vi "lvCopy.vi"(8 "error in (no error)":errorcluster, 11 "CommandLine":string[](array[string])) -> (0 "error out":errorcluster, 2 "test details":string, 3 "output to action":string)   [LabVIEW 2014]
uses:
  <userlib>/_OpenG.lib/file/file.llb/Build Path - File Names Array__ogtk.vi
  _lvcicd/_lvcicd_support_2014.lvlib
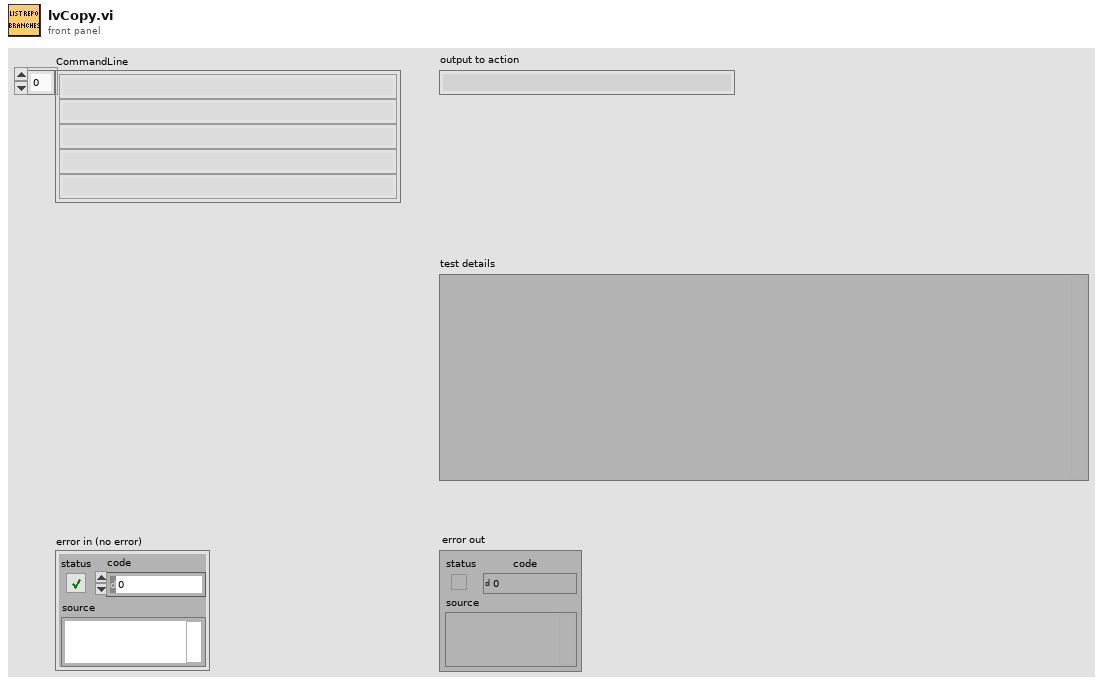
[diagram p1: front panel]
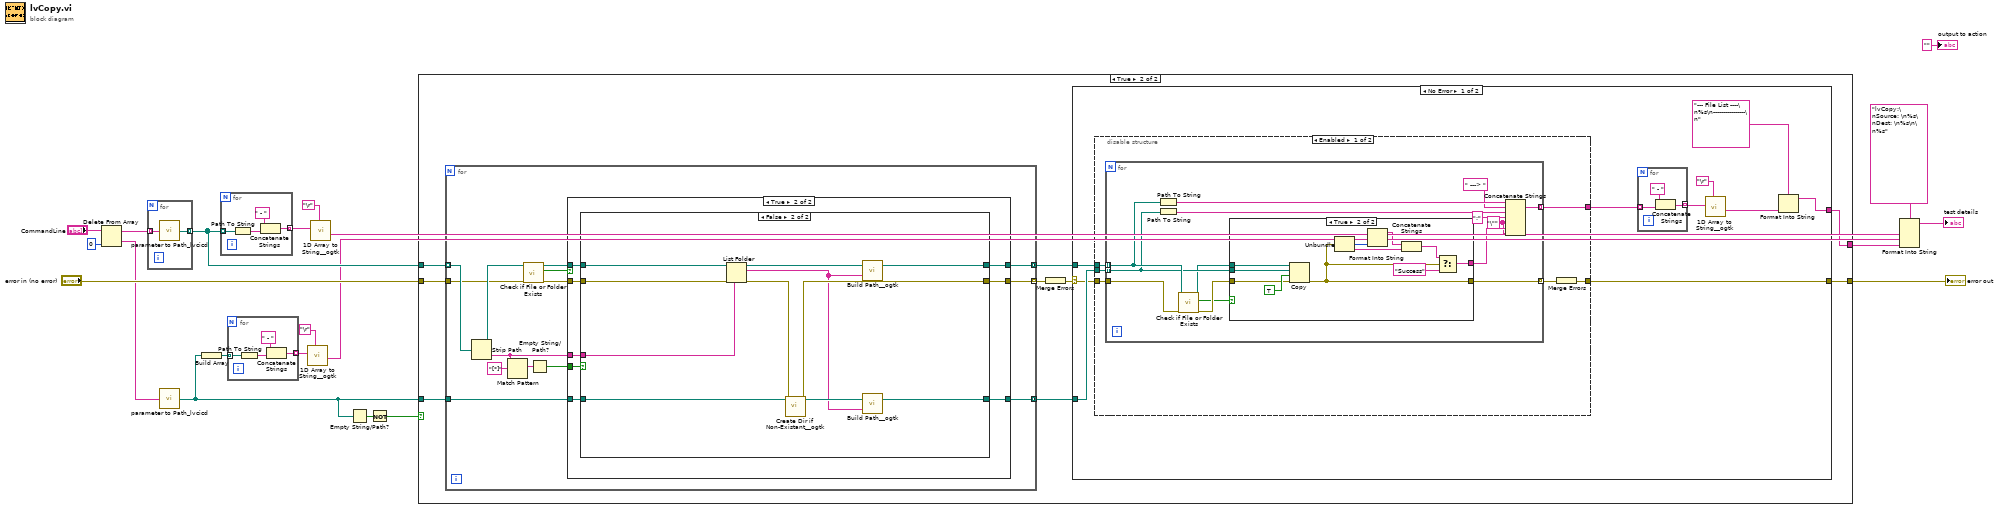
[diagram p0: block diagram]
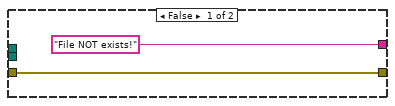
[diagram p3: hidden frame]
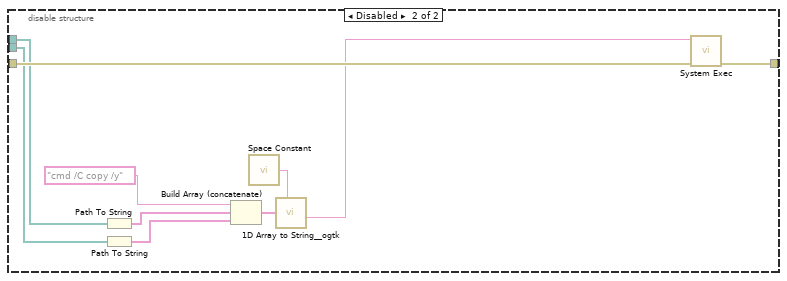
[diagram p4: hidden frame]
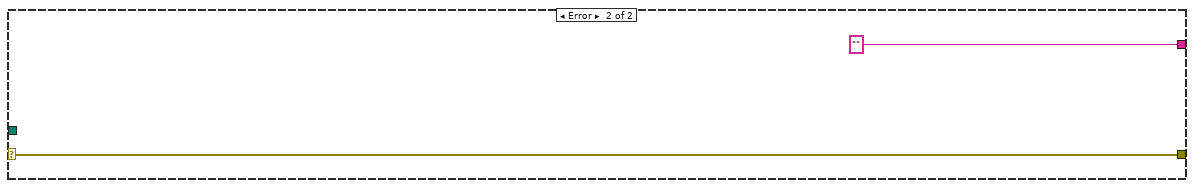
[diagram p5: hidden frame]
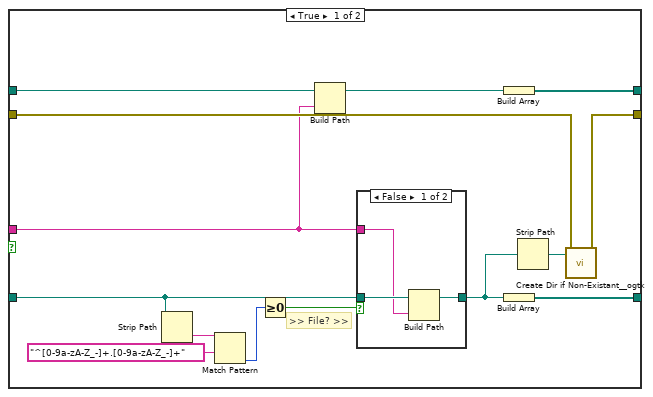
[diagram p7: hidden frame]
diagram:
  n1 = Delete From Array(array="CommandLine", index=0) -> (deleted portion=w13:string, array with subset deleted=w12:string[])  [unwired: 1 in]
  n2 = for {
    tunnel: [w23] -> w11 mode=indexing
    tunnel: w12 -> [w22] mode=indexing
    n3 = call "parameter to Path_lvcicd.vi"("String"=w22) -> ("Path"=w23:path)
  }
  n4 = call "parameter to Path_lvcicd.vi"("String"=w13) -> ("Path"=w3:path)
  n5 = Build Array(w3) -> (w4:path[])
  n6 = for {
    tunnel: w11 -> [w27] mode=indexing
    tunnel: [w24] -> w10 mode=indexing
    n7 = Path To String(path=w27) -> (string=w26:string)
    n8 = Concatenate Strings(" - " ("string"), w26) -> (w24:string)
  }
  n9 = for {
    tunnel: w4 -> [w31] mode=indexing
    tunnel: [w28] -> w5 mode=indexing
    n10 = Path To String(path=w31) -> (string=w30:string)
    n11 = Concatenate Strings(" - " ("string"), w30) -> (w28:string)
  }
  n12 = call <userlib>:"1D Array to String__ogtk.vi"("delimiter (Tab)"="\r", "Array of Strings"=w5) -> ("delimited string"=w2:string)  [unwired: 9 in]
  n13 = call <userlib>:"1D Array to String__ogtk.vi"("delimiter (Tab)"="\r", "Array of Strings"=w10) -> ("delimited string"=w8:string)  [unwired: 9 in]
  n14 = Empty String/Path?(string/path=w3) -> (empty?=w20:bool)
  n15 = Not(x=w20) -> (.not. x?=w18:bool)
  n16 = case shown="True" w18 {
    tunnel: "error in (no error)" -> [w32 w41]
    tunnel: [w32 w40] -> w21
    tunnel: w11 -> [_ w39]
    tunnel: w3 -> [_ w38]
    tunnel: [_ w37] -> w7
    frame False {
    }
    frame True {
      n17 = for {
        tunnel: w39 -> [w113] mode=indexing
        tunnel: w38 -> [w112]
        tunnel: [w105] -> w35 mode=concatenating
        tunnel: [w104] -> w34 mode=concatenating
        tunnel: w41 -> [w102]
        tunnel: [w106] -> w36 mode=indexing
        n18 = Strip Path(path=w113) -> (stripped path=w107:path, name=w111:string)
        n19 = Match Pattern(string=w111, regular expression="[*]") -> (match substring=w109:string)  [unwired: 1 in, 3 out]
        n20 = call <vilib>:"Check if File or Folder Exists.vi"("error in (no error)"=w102, "path"=w107) -> ("error out"=w101:errorcluster, "file or folder exists?"=w100:bool, "dup path"=w103:path)  [unwired: 7 in]
        n21 = Empty String/Path?(string/path=w109) -> (empty?=w108:bool)
        n22 = case shown="True" w100 {
          tunnel: w112 -> [_ w122]
          tunnel: w111 -> [_ w121]
          tunnel: w108 -> [_ w120]
          tunnel: [w114 w119] -> w106
          tunnel: [_ w118] -> w105
          tunnel: [_ w117] -> w104
          tunnel: w103 -> [_ w116]
          tunnel: w101 -> [w114 w115]
          frame False {
          }
          frame True {
            n23 = case shown="False" w120 {
              tunnel: w122 -> [w127 w147]
              tunnel: [w136 w150] -> w118
              tunnel: w121 -> [w130 w151]
              tunnel: w116 -> [w131 w146]
              tunnel: w115 -> [w133 w145]
              tunnel: [w132 w149] -> w119
              tunnel: [w128 w148] -> w117
              frame True {
                # ">> File? >>"
                n24 = Strip Path(path=w127) -> (name=w126:string)  [unwired: 1 out]
                n25 = Match Pattern(string=w126, regular expression="^[0-9a-zA-Z_-]+.[0-9a-zA-Z_-]+") -> (offset past match=w123:i32)  [unwired: 1 in, 3 out]
                n26 = Greater Or Equal To 0?(x=w123) -> (x >= 0?=w124:bool)
                n27 = Build Path(base path=w131, name or relative path=w130) -> (appended path=w129:path)
                n28 = case shown="False" w124 {
                  tunnel: w127 -> [w139 w140]
                  tunnel: [w138 w140] -> w134
                  tunnel: w130 -> [w137 _]
                  frame False {
                    n29 = Build Path(base path=w139, name or relative path=w137) -> (appended path=w138:path)
                  }
                  frame True {
                  }
                }
                n30 = Build Array(w129) -> (w128:path[])
                n31 = Build Array(w134) -> (w136:path[])
                n32 = Strip Path(path=w134) -> (stripped path=w135:path)  [unwired: 1 out]
                n33 = call <userlib>:"Create Dir if Non-Existant__ogtk.vi"("error in (no error)"=w133, "Directory Path"=w135) -> ("error out"=w132:errorcluster)  [unwired: 7 in, 2 out]
              }
              frame False {
                n34 = List Folder(path=w146, pattern=w151, error in=w145) -> (path out=w142:path, filenames=w141:string[], error out=w143:errorcluster)  [unwired: 1 in, 1 out]
                n35 = call <userlib>:"Create Dir if Non-Existant__ogtk.vi"("error in (no error)"=w143, "Directory Path"=w147) -> ("error out"=w149:errorcluster, "dup Directory Path"=w144:path)  [unwired: 7 in, 1 out]
                n36 = call-poly <userlib>:"Build Path__ogtk.vi"("name or relative path"=w141, "base path"=w142) -> ("appended path"=w148:path[])
                n37 = call-poly <userlib>:"Build Path__ogtk.vi"("name or relative path"=w141, "base path"=w144) -> ("appended path"=w150:path[])
              }
            }
          }
        }
      }
      n38 = Merge Errors(w36) -> (w33:errorcluster)
      n39 = case shown="No Error" w33 {
        selector: w33 -> [w45 w99]
        tunnel: [w51 w99] -> w40
        tunnel: [w42 "" ("delimited string")] -> w37
        tunnel: w35 -> [w47 _]
        tunnel: w34 -> [w46 _]
        frame No Error {
          n40 = disable-structure shown="Enabled" {
            disable-tunnel: w45 -> [w57 w93]
            disable-tunnel: [w53 w94] -> w51
            disable-tunnel: w47 -> [w55 w91]
            disable-tunnel: w46 -> [w54 w92]
            disable-tunnel: [w52 _] -> w48
            frame Enabled {
              n41 = for {
                tunnel: w55 -> [w65] mode=indexing
                tunnel: w54 -> [w66] mode=indexing
                tunnel: w57 -> [w63]
                tunnel: [w71] -> w56 mode=indexing
                tunnel: [w70] -> w52 mode=indexing
                w58 = "\"" ("string")
                n42 = Path To String(path=w66) -> (string=w69:string)
                n43 = Path To String(path=w65) -> (string=w68:string)
                n44 = call <vilib>:"Check if File or Folder Exists.vi"("error in (no error)"=w63, "path"=w66) -> ("error out"=w62:errorcluster, "file or folder exists?"=w61:bool, "dup path"=w64:path)  [unwired: 7 in]
                n45 = case shown="True" w61 {
                  tunnel: [w73 w78] -> w71
                  tunnel: w65 -> [_ w83]
                  tunnel: w64 -> [_ w82]
                  tunnel: w62 -> [w73 w81]
                  tunnel: ["File NOT exists!" ("string") w80] -> w59
                  frame False {
                  }
                  frame True {
                    n46 = Copy(8:w81, 9:TRUE ("overwrite (F)"), 10:w83, 11:w82) -> (0:w78:errorcluster)  [unwired: 1 in, 2 out]
                    n47 = Unbundle(w78) -> ("code"=w76:i32, "source"=w77:string)  [unwired: 1 out]
                    n48 = Format Into String(w76) -> (resulting string=w75:string)  [unwired: 3 in, 1 out]
                    n49 = Concatenate Strings(w75, w77) -> (w74:string)
                    n50 = Select(t=w74, s=w78, f="Success" ("string")) -> (s? t:f=w80:string)
                  }
                }
                n51 = Concatenate Strings(w69, " ---> " ("string"), w68, ":" ("string"), w58, w59, w58) -> (w70:string)
              }
              n52 = Merge Errors(w56) -> (w53:errorcluster)
            }
            frame Disabled {
              n53 = Path To String(path=w92) -> (string=w89:string[])
              n54 = Path To String(path=w91) -> (string=w88:string[])
              n55 = Build Array (concatenate)("cmd /C copy /y" ("name"), w89, w88) -> (w87:string[])
              n56 = call <vilib>:"Space Constant.vi"() -> ("String"=w86:string)
              n57 = call <userlib>:"1D Array to String__ogtk.vi"("delimiter (Tab)"=w86, "Array of Strings"=w87) -> ("delimited string"=w85:string)  [unwired: 9 in]
              n58 = call <vilib>:"System Exec.vi"("error in (no error)"=w93, "command line"=w85) -> ("error out"=w94:errorcluster)  [unwired: 6 in, 3 out]
            }
          }
          n59 = for {
            tunnel: [w96] -> w50 mode=indexing
            tunnel: w48 -> [w95] mode=indexing
            n60 = Concatenate Strings(" - " ("string"), w95) -> (w96:string)
          }
          n61 = call <userlib>:"1D Array to String__ogtk.vi"("delimiter (Tab)"="\r", "Array of Strings"=w50) -> ("delimited string"=w43:string)  [unwired: 9 in]
          n62 = Format Into String(format string="--- File List ----\n%s\n----------------\n", w43) -> (resulting string=w42:string)  [unwired: 2 in, 1 out]
        }
        frame Error {
        }
      }
    }
  }
  "error out" <- w21
  n63 = Format Into String(format string="lvCopy:\nSource: \n%s\nDest: \n%s\n\n%s", w8, w2, w7) -> (resulting string=→"test details":string)  [unwired: 2 in, 1 out]
  "output to action" <- "" ("output to action")
